vi "Switch Cal Standard.vi"(0 "ACM4509 in":refnum<class "Cal Standard.lvclass">, 5 "Standard Type":T1, 7 "Path Name":string, 11 "error in (no error)":errorcluster) -> (4 "ACM4509 out":refnum<class "Cal Standard.lvclass">, 15 "error out":errorcluster)   [LabVIEW 2023, in "ACM 4509 Cal Standard.lvlib" / "Cal Standard.lvclass"]
uses:
  Cal Standard.lvclass
  Instruments/Cal Standard/Type Definitions/Standard Type.ctl
  Cal Standard.lvclass/Cal Standard.ctl
  Properties/Read Resource Name.vi
  Properties/Read Product Name.vi
  Dependencies/ACM/ACM Visa Driver.lvlib
  Common/RFCalAndFixtureCharact.Common.lvlib
  Instruments/RFFixtureCharact.Instruments.lvlib
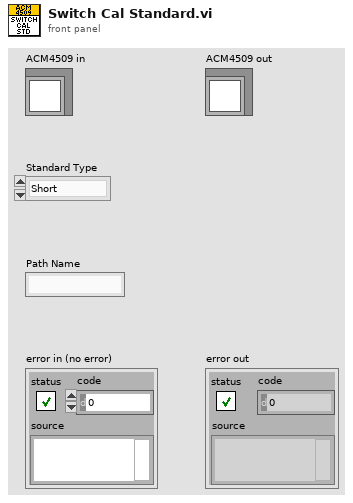
[diagram p1: front panel]
types:
  T1 = typedef "RFFixtureCharact.Instruments.lvlib/Standard Type.ctl" = enum16{"Short", "Open", "Load"}
  T2 = typedef "ACM Visa Driver.lvlib/ACM Switch States.ctl" = string
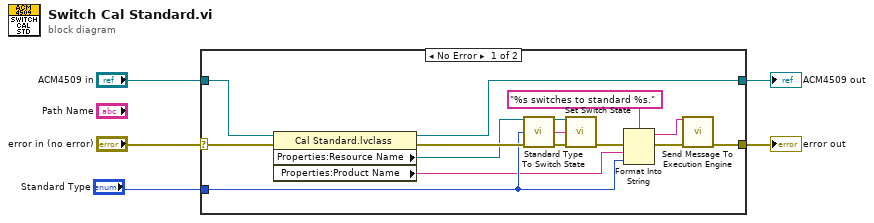
[diagram p0: block diagram]
diagram:
  n1 = case shown="No Error" "error in (no error)" {
    selector: "error in (no error)" -> [w15 w20]
    tunnel: [w9 w20] -> w2
    tunnel: [w13 w19] -> w4
    tunnel: "ACM4509 in" -> [w14 w19]
    tunnel: "Standard Type" -> [w7 _]
    frame No Error {
      n2 = property class="Cal Standard.lvclass"(reference=w14, error in=w15) -> (reference out=w13:refnum<class "Cal Standard.lvclass">, error out=w17:errorcluster, "Properties:Resource Name"=w16:refnum<visa-resource-name>, "Properties:Product Name"=w6:string)
      n3 = call "Standard Type To Switch State.vi"("Standard Type"=w7) -> ("Switch State"=w18:T2)
      n4 = call "Set Switch State.vi"("VISA resource name"=w16, "Switch State"=w18, "error in (no error)"=w17) -> ("error out"=w10:errorcluster)  [unwired: 11 in, 1 out]
      n5 = Format Into String(format string="%s switches to standard %s." ("message"), error in=w10, w6, w7) -> (resulting string=w11:string, error out=w12:errorcluster)  [unwired: 1 in]
      n6 = call "Send Message To Execution Engine.vi"("Message"=w11, "error in (no error)"=w12) -> ("error out"=w9:errorcluster)  [unwired: 13 in]
    }
    frame Error {
    }
  }
  "error out" <- w2
  "ACM4509 out" <- w4
